vi "FxPlateCoords.vi"(9 "Array":string[](array[string]), 10 "Subject Name":string, 11 ".NET Refnum in":refnum<k24>) -> (3 "Translation":dbl[][](array[numeric]))   [LabVIEW 2013]
uses:
  D:/TPAD/Dropbox/LabviewStuff/activeTPAD_LV/Vicon_files/ViconDataStreamSDK_DotNET.dll
  Vicon_files/ViconDataStreamSDK_DotNET.dll
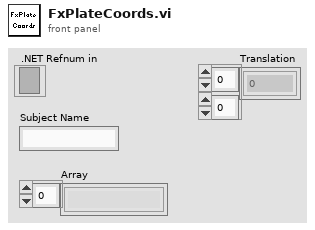
[diagram p1: front panel]
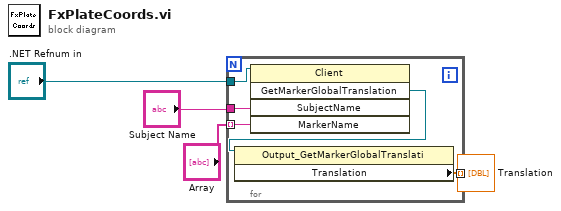
[diagram p0: block diagram]
diagram:
  n1 = for {
    tunnel: "Subject Name" -> [w8]
    tunnel: [w7] -> w1 mode=indexing
    tunnel: ".NET Refnum in" -> [w6]
    tunnel: "Array" -> [w5] mode=indexing
    n2 = invoke class="Client" method="GetMarkerGlobalTranslation"(reference=w6, "SubjectName"=w8, "MarkerName"=w5) -> ("GetMarkerGlobalTranslation"=w9:refnum<k24>)  [unwired: 2 in, 4 out]
    n3 = property class="Output_GetMarkerGlobalTranslati"(reference=w9) -> ("Translation"=w7:dbl[])  [unwired: 1 in, 2 out]
  }
  "Translation" <- w1
